vi "Shutdown.vi"(8 "error in":errorcluster, 11 "CrossPoint in":refnum<class "CrossPoint.lvclass">) -> (0 "error out":errorcluster, 3 "CrossPoint out":refnum<class "CrossPoint.lvclass">)   [LabVIEW 2019, in "CrossPoint.lvlib" / "CrossPoint.lvclass"]
uses:
  Library/CrossPoint.lvclass
  builds/Instruments/Instruments.lvlibp/Library/Instruments.lvclass
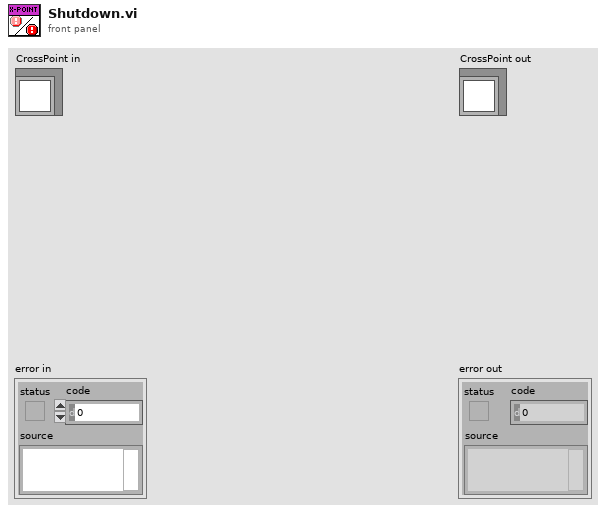
[diagram p1: front panel]
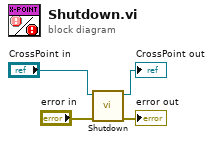
[diagram p0: block diagram]
diagram:
  n1 = call-parent "Shutdown.vi"("error in"="error in", "Instruments in"="CrossPoint in") -> ("error out"=→"error out":errorcluster, "Instruments out"=→"CrossPoint out":refnum<class "CrossPoint.lvclass">)  [unwired: 8 in]
